vi "Close (SubVI for PI).vi"   [LabVIEW 2020]
uses:
  Global Parameters.vi
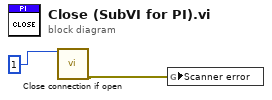
[diagram p0: block diagram]
diagram:
  n1 = call "Close connection if open.vi"("System no."=1) -> ("error out"=w1:errorcluster)  [unwired: 2 in, 16 out]
  n2 = global write "Global Parameters.vi" "Scanner error"(w1) -> ()
